vi "poc.ip.kria.vi"(0 "ip.reset":bool, 1 "TDATA":u64, 2 "TKEEP":u8, 3 "TUSER":bool, 4 "TVALID":bool, 5 "TLAST":bool, 6 "DEBUG.TREADY":bool, 7 "CMD.TREADY":bool, 9 "MDEBUG.TREADY":bool) -> ()   [LabVIEW 2020]
uses:
  <vilib>/Platform/TimedLoop/XDataNode/timing_clust.ctl
  <vilib>/Platform/TimedLoop/XDataNode/nitl_modes.ctl
  <vilib>/Platform/TimedLoop/XDataNode/wakeup.ctl
  submodules/Market.Data.Common/fpga/my.network.data.stream.ctl
  submodules/Market.Data.Bats.Parser/fpga/poc.ip.debug.states.ctl
  submodules/Market.Data.Common/fpga/orderbook.command.ctl
  submodules/Market.Data.Common/fpga/orderbook.command.type.ctl
  submodules/Market.Data.Bats.Parser/fpga/poc.ip.axi.write.states.ctl
  <instrlib>/_niInstr/Network/Types/v1/IPv4 Address.ctl
  <instrlib>/_niInstr/Network/Types/v1/MAC Address.ctl
  Ethernet MAC - Custom/Ethernet MAC - Custom.lvclass
  axi_2_eth_raw.ctl
  <vilib>/rvi/DataTransferAndStorage/Container/Common/niFpgaContainerGetUniqueNameForEmu.vi
  <vilib>/rvi/DataTransferAndStorage/Container/Common/niFpgaContainerSetEmuInfo.vi
  <vilib>/rvi/eio/common/nirviEmuReportErrorAndStop.vi
  <vilib>/rvi/Emulation/niFpgaSctlEmulationGetInTimedLoop.vi
  <vilib>/rvi/Emulation/niFpgaEmulationReportErrorSimple.vi
  <vilib>/rvi/Emulation/niFpgaGetClockAttributes.vi
  <vilib>/rvi/Emulation/niFpgaCriticalErrorInLSC.vi
  <vilib>/rvi/Emulation/niFpgaEmulationIsFPGAContextNoSignature.vi
  <vilib>/rvi/errors/niFpgaSetErrorForExecOnDevCompSimple.vi
  <vilib>/rvi/FIFO/Fifo_Resource/nirvififoEmulationSetSize.vi
  <vilib>/rvi/FIFO/Fifo_Resource/nirviFifoEmulationQueueMgr.vi
  <instcachedir>/0/nirviFifoEmulationQueueMgr_E5CAEC123FF24DC58D834DCA3CDAA9B5.lvgen/nirviFifoEmulationQueueMgr_E5CAEC123FF24DC58D834DCA3CDAA9B5_017.vi
  <vilib>/Utility/error.llb/Clear Errors.vi
  <vilib>/rvi/FIFO/Fifo_Resource/nirvififoEmulationCreateLock.vi
  <vilib>/rvi/Emulation/niFpgaProcessEmulError.vi
  <vilib>/rvi/FIFO/Fifo_Resource/nirvififoEmulationObtainLock.vi
  <vilib>/rvi/FIFO/Fifo_Resource/nirvififoEmulationReleaseLock.vi
  <vilib>/rvi/occurrence/nirviWaitOnOccurrenceBase.vi
  <vilib>/rvi/errors/nirviReportUnexpectedCaseInternalError.vi
  <vilib>/rvi/errors/nirviReportUnexpectedCaseInternalError (U32).vi
  <vilib>/rvi/interface/RandomDataEmulation/nirviRandomDataMultiElementFPGAFIFO.vi
  <instcachedir>/0/nirviRandomDataMultiElementFPGAFIFO_3E9965BA1FAD4E7B8DABA31768A09B1F.lvgen/nirviRandomDataMultiElementFPGAFIFO_3E9965BA1FAD4E7B8DABA31768A09B1F_001.vi
  <vilib>/rvi/interface/RandomDataEmulation/niFpgaRandomDataHandleErrors.vi
  <instcachedir>/0/nirviFifoEmulationQueueMgr_E5CAEC123FF24DC58D834DCA3CDAA9B5.lvgen/nirviFifoEmulationQueueMgr_E5CAEC123FF24DC58D834DCA3CDAA9B5_020.vi
  <vilib>/rvi/DataTransferAndStorage/Container/Common/niFpgaContainerExecOnDevCompGetState.vi
  <vilib>/rvi/Memory/Memory_Emulation/niFpgaMemoryEmulationCacheClearOnFirstRun.vi
  <vilib>/rvi/Memory/Memory_Emulation/nirvimemoryEmulationManagerCache_MakeExclusive.vi
  <vilib>/rvi/Memory/Memory_Emulation/niFpgaMemoryEmulationValidateCache.vi
  <vilib>/rvi/Memory/Memory_Emulation/nirvimemoryEmulationManagerCache_InsertValue.vi
  <vilib>/rvi/Memory/Memory_Emulation/nirvimemoryEmulationManagerCache_ReleaseExclusive.vi
  <vilib>/rvi/Memory/Memory_Emulation/nirvimemoryEmulationManagerCache_GetValue.vi
  <vilib>/rvi/Memory/Memory_Emulation/nirvimemoryEmulationManagerCache_SetValue.vi
  <instcachedir>/0/nirviFifoEmulationQueueMgr_E5CAEC123FF24DC58D834DCA3CDAA9B5.lvgen/nirviFifoEmulationQueueMgr_E5CAEC123FF24DC58D834DCA3CDAA9B5_021.vi
  <vilib>/rvi/FIFO/Fifo_Resource/nirvififoEmulationDetermineInputValidOut.vi
  <instcachedir>/0/nirviFifoEmulationQueueMgr_E5CAEC123FF24DC58D834DCA3CDAA9B5.lvgen/nirviFifoEmulationQueueMgr_E5CAEC123FF24DC58D834DCA3CDAA9B5_018.vi
  <vilib>/rvi/Emulation/niFpgaSctlEmulationResourceMgr.vi
  <instrlib>/_niInstr/Network/IPv4/Data Stream/v1/Read IPv4 Header.vi
  <instrlib>/_niInstr/Network/IPv4/UDP/Data Stream/v1/Read End of Bad Frame.vi
  <instrlib>/_niInstr/Network/IPv4/UDP/Data Stream/v1/Read End of Good Frame.vi
  <instrlib>/_niInstr/Network/IPv4/UDP/Data Stream/v1/Read Data Stream.vi
  <vilib>/Platform/TimedLoop/XDataNode/XDataNode.xnode
  <vilib>/rvi/LocalResourceManager/LocalResourceManager.xnode
  <vilib>/rvi/DataTransferAndStorage/Container/XNode/niFpgaContainer.xnode
  <vilib>/rvi/FIFO/Fifo_Resource/nirvififoEmulationRead.vi
  <vilib>/rvi/interface/RandomDataEmulation/nirviRandomDataFpgaMultiElementTemplate.vi
  <vilib>/rvi/DataTransferAndStorage/Register/Emulation/niFpgaRegisterEmulationRefIn.vi
  <vilib>/rvi/FIFO/Fifo_Resource/niFpgaFifoEmulationRefIn.vi
  <vilib>/rvi/Memory/Memory_Emulation/niFpgaMemoryEmulationRefIn.vi
  <vilib>/rvi/FIFO/Fifo_Resource/nirvififoEmulationWrite.vi
  <vilib>/Platform/TimedLoop/XDataNode/XDNodeRunTimeDep.lvlib
  submodules/Market.Data.Common/fpga/fpganow.common.fpga.lvlib
  <instrlib>/_niInstr/Network/IPv4/UDP/Data Stream/v1/niInstr IPv4 UDP Data Stream v1.lvclass
  <instrlib>/_niInstr/Network/Ethernet/Utility/v1/FPGA/niInstr Ethernet Utilities FPGA v1.lvlib
  <instrlib>/_niInstr/Network/IPv4/FPGA/v1/niInstr IPv4 FPGA v1.lvlib
  <instrlib>/_niInstr/Network/IPv4/UDP/FPGA/v1/niInstr IPv4 UDP FPGA v1.lvlib
  <instrlib>/_niInstr/Network/Types/v1/niInstr Network Types v1.lvlib
  <instrlib>/_niInstr/Network/IPv4/Data Stream/v1/niInstr IPv4 Data Stream v1.lvclass
panel:
  out "MDEBUG.TLAST":bool
  out "MDEBUG.TVALID":bool
  out "MDEBUG.TKEEP":u8
  out "MDEBUG.TDATA":u64
  out "CMD.TKEEP":u8
  out "CMD.TDATA":u64
  out "CMD.TLAST":bool
  out "CMD.TVALID":bool
  out "DEBUG.TLAST":bool
  out "DEBUG.TVALID":bool
  out "DEBUG.TKEEP":u8
  out "DEBUG.TDATA":u64
  # "This VI will be IP Exported"
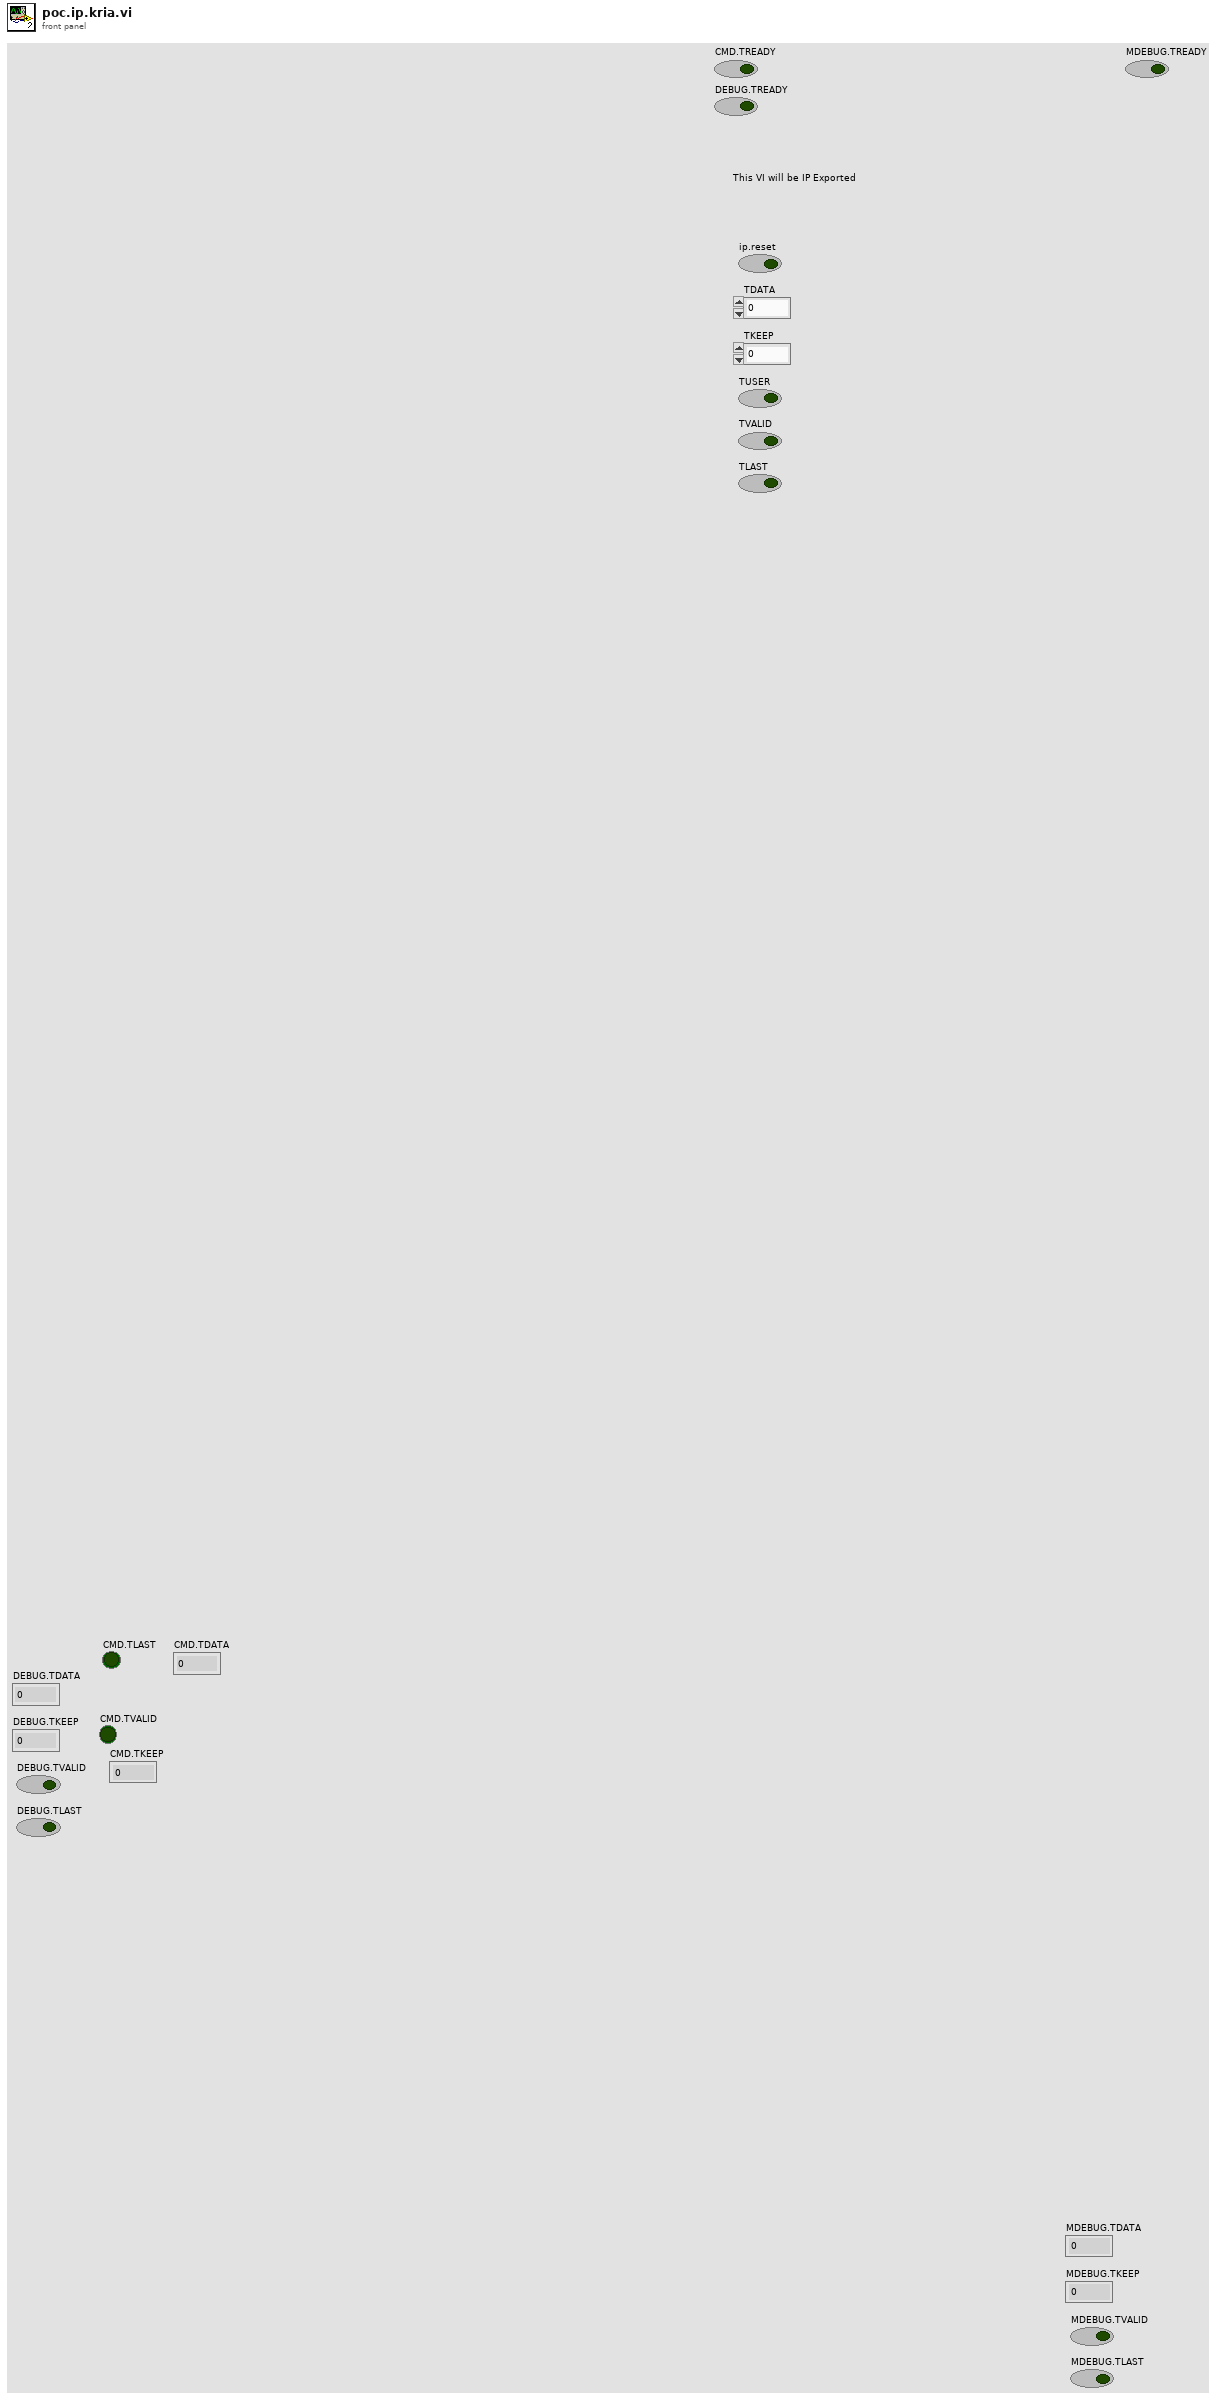
[diagram p1: front panel]
types:
  T1 = typedef "XDNodeRunTimeDep.lvlib/timing_clust.ctl" = cluster{"Expected End [f-1]":u64, "Actual End [f-1]":u64, "Finished Late? [f-1]":bool, "Expected End [i-1]":u64, "Actual End [i-1]":u64, "Finished Late? [i-1]":bool, "Expected Start [i]":u64, "Actual Start [i]":u64, "Expected Start [f]":u64, "Actual Start [f]":u64, "Source Name":string, "Structure Name":string, "Period":i64, "Deadline":i64, "Offset":i64, "Start":i64, "Priority":i32, "Timeout":i32, "Mode":T2, "Wakeup Reason":T3, "Error":errorcluster, "Source Type":string, "Secondary Source Type":string, "Global End Time":u64, "Global Start Time":u64, "Frame Duration":u64, "Iteration Duration":u64, "Assigned CPU":i32, "I/O Scan Engine Mode":u32}
  T2 = typedef "XDNodeRunTimeDep.lvlib/nitl_modes.ctl" = enum32{"No Change", "Process missed periods, maintain original phase", "Discard missed periods, maintain original phase", "Process missed periods, ignore original phase", "Discard missed periods, ignore original phase"}
  T3 = typedef "XDNodeRunTimeDep.lvlib/wakeup.ctl" = enum32{"Normal", "Aborted", "Asynchronous wakeup", "Timing source error", "Timed loop error", "Timeout"}
  T4 = typedef "niInstr Network Types v1.lvlib/MAC Address.ctl" = u8[]
  T5 = typedef "niInstr Network Types v1.lvlib/IPv4 Address.ctl" = u8[]
  T6 = typedef "my.network.data.stream.ctl" = cluster{"data":u8[], "data valid":bool, "byte enables":bool[], "eof.good":bool, "eof.bad":bool, "frame.start":u64}
  T7 = cluster{"TDATA":u64, "TKEEP":u8, "TVALID":bool, "TLAST":bool, "TUSER":bool}
  T8 = cluster{"data valid":bool, "end.of.frame":bool, "start.of.frame":bool, "data":u64, "byte enables":u8}
  T9 = typedef "axi_2_eth_raw.ctl" = cluster{"data valid":bool, "end.of.frame":bool, "start.of.frame":bool, "data":u64, "byte enables":u8}
  T10 = typedef "niInstr IPv4 FPGA v1.lvlib/IPv4 Header.ctl" = cluster{"Version":fxp<+,4,4>, "IHL":fxp<+,4,4>, "DSCP":fxp<+,6,6>, "ECN":fxp<+,2,2>, "Total Length":u16, "Identification":u16, "Flags":fxp<+,3,3>, "Fragment Offset":fxp<+,13,13>, "Time To Live":u8, "Protocol":T11, "Header Checksum":u16, "Source IP":u8[], "Dest IP":u8[]}
  T11 = typedef "niInstr IPv4 FPGA v1.lvlib/IPv4 Protocols.ctl" = u8
  T12 = typedef "niInstr Ethernet Utilities FPGA v1.lvlib/Network Data Stream.ctl" = cluster{"data":u8[], "data valid":bool, "byte enables":bool[]}
  T13 = typedef "poc.ip.debug.states.ctl" = enum16{"Wait", "Write.Data"}
  T14 = typedef "poc.ip.axi.write.states.ctl" = enum16{"Wait", "Collect"}
  T15 = typedef "fpganow.common.fpga.lvlib/orderbook.command.ctl" = cluster{"type":T16, "side":u8, "orderId ":u64, "quantity":u32, "symbol":u64, "price":u64, "executed.qty":u32, "canceled.qty":u32, "remaining.qty":u32, "seconds":u64, "nanoseconds":u64, "Add":bool, "Edit":bool, "Remove":bool, "seq no":u32, "recv.time":u64, "parse.time":u64}
  T16 = typedef "fpganow.common.fpga.lvlib/orderbook.command.type.ctl" = enum8{"Time", "AddOrder", "OrderExecuted", "OrderExecutedAtPrice", "ReduceSize", "ModifyOrder", "DeleteOrder", "Get.Everything", "Get.All.Orders", "Get.Top"}
  T17 = cluster{"state":T13, "ob.cmd":T15, "index":i16, "TLAST":bool, "TDATA":u64}
  T18 = cluster{"state":T13, "arr":u64[], "index":u8, "TLAST":bool, "TDATA":u64}
  T19 = cluster{"type":enum8{"Time", "AddOrder", "OrderExecuted", "OrderExecutedAtPrice", "ReduceSize", "ModifyOrder", "DeleteOrder", "Get.Everything", "Get.All.Orders", "Get.Top"}, "side":u8, "orderId ":u64, "quantity":u32, "symbol":u64, "price":u64, "executed.qty":u32, "canceled.qty":u32, "remaining.qty":u32, "seconds":u64, "nanoseconds":u64, "Add":bool, "Edit":bool, "Remove":bool, "seq no":u32, "recv.time":u64, "parse.time":u64}
  T20 = enum8{"Time", "AddOrder", "OrderExecuted", "OrderExecutedAtPrice", "ReduceSize", "ModifyOrder", "DeleteOrder", "Get.Everything", "Get.All.Orders", "Get.Top"}
  T21 = cluster{"data":u8[], "data valid":bool, "byte enables":bool[], "eof.good":bool, "eof.bad":bool, "Timestamp":u64}
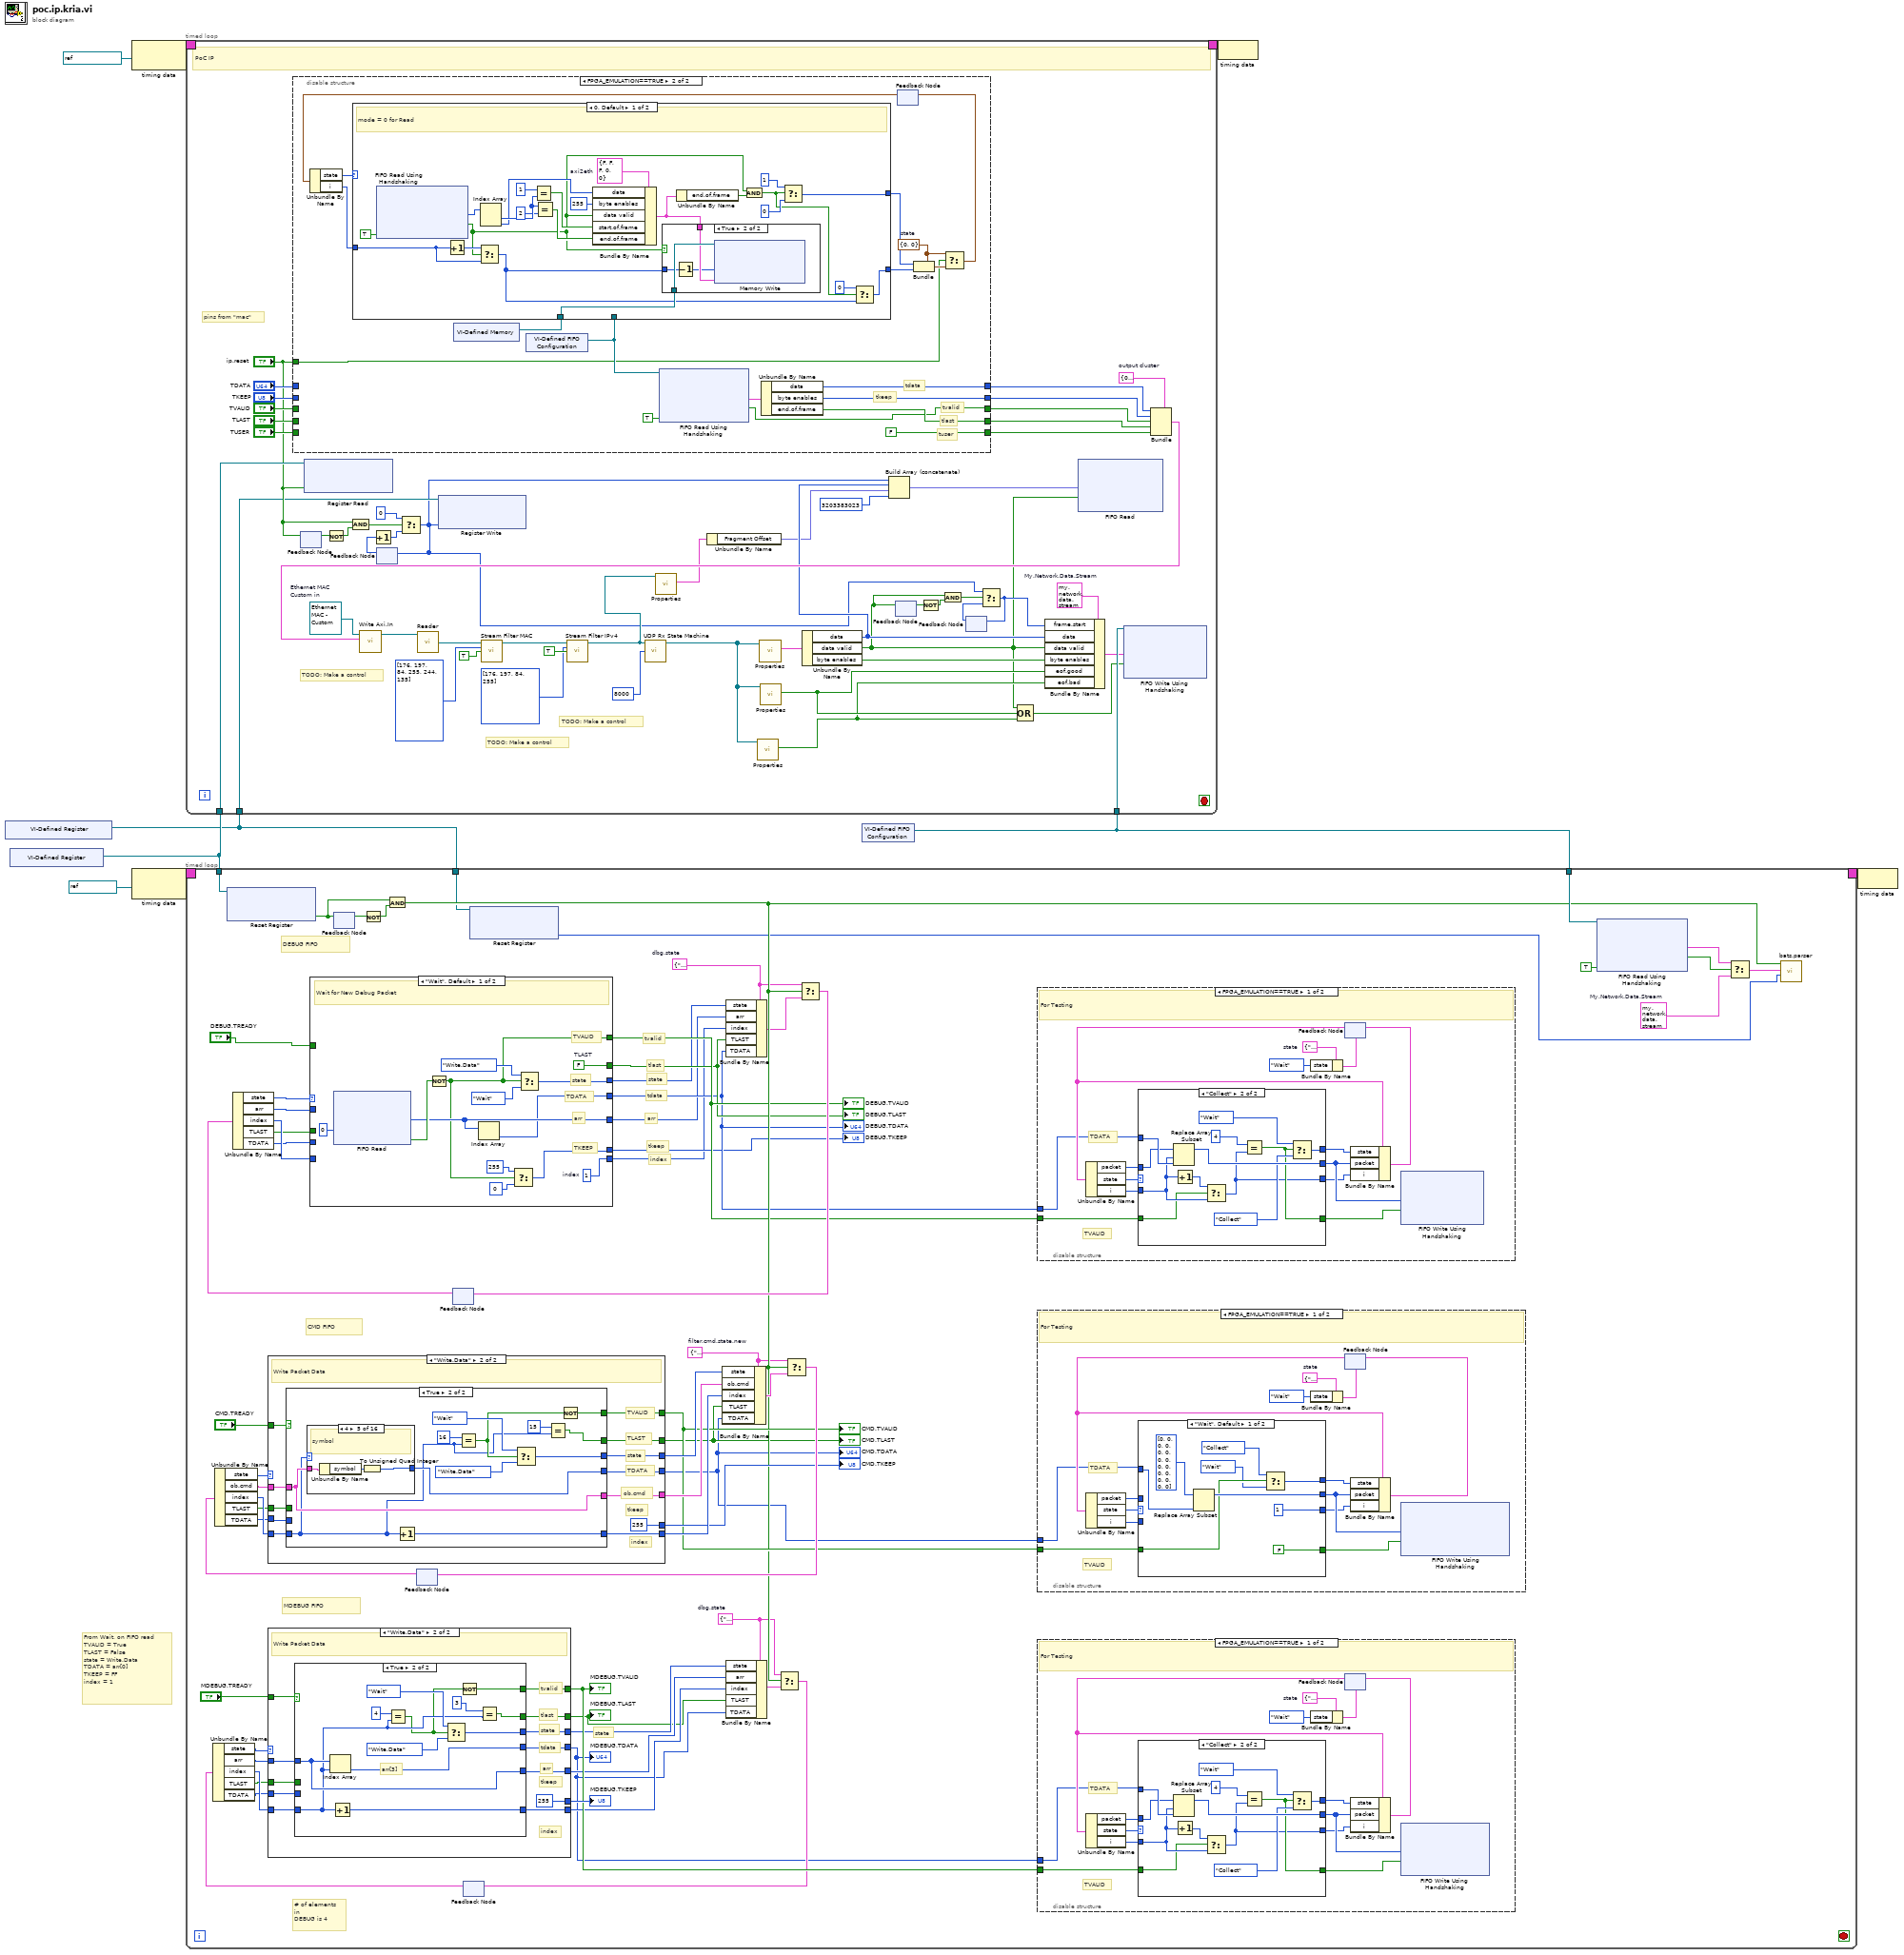
[diagram p0: block diagram]
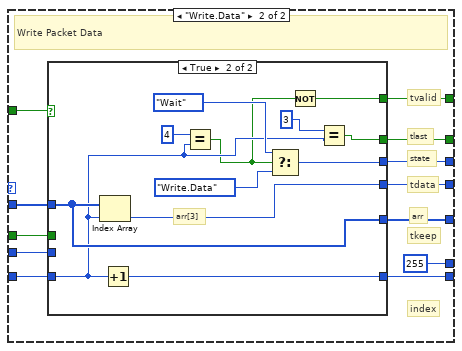
[diagram p2: hidden frame]
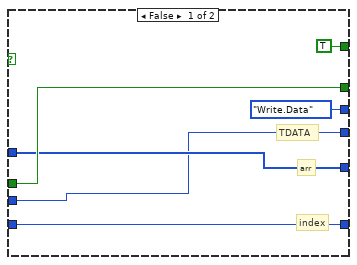
[diagram p3: hidden frame]
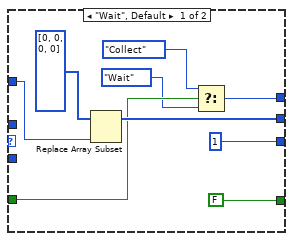
[diagram p4: hidden frame]
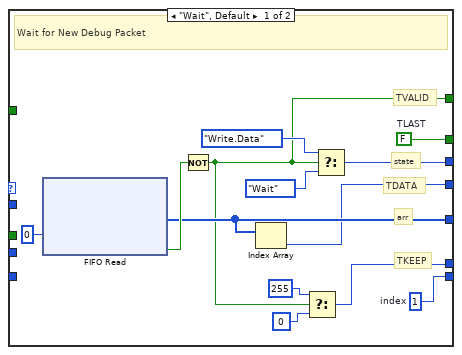
[diagram p6: hidden frame]
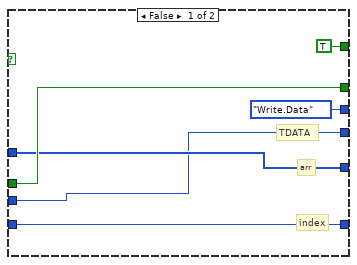
[diagram p7: hidden frame]
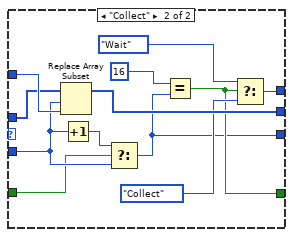
[diagram p8: hidden frame]
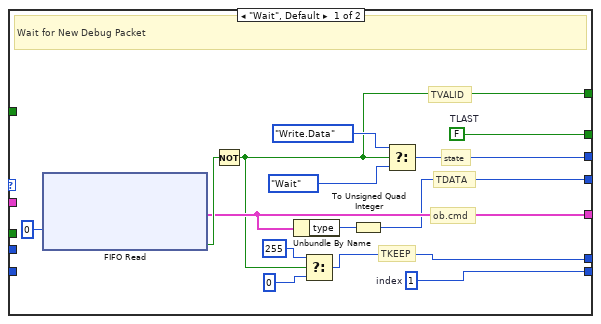
[diagram p10: hidden frame]
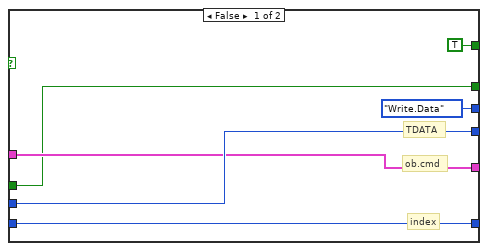
[diagram p11: hidden frame]
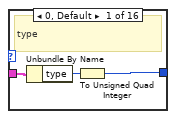
[diagram p12: hidden frame]
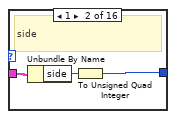
[diagram p13: hidden frame]
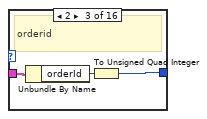
[diagram p14: hidden frame]
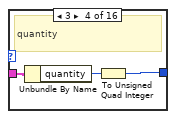
[diagram p15: hidden frame]
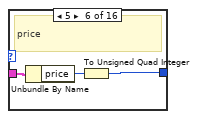
[diagram p16: hidden frame]
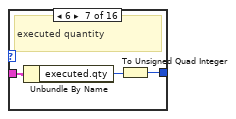
[diagram p17: hidden frame]
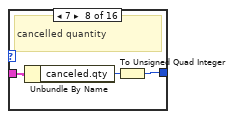
[diagram p18: hidden frame]
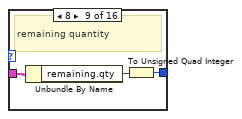
[diagram p19: hidden frame]
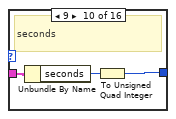
[diagram p20: hidden frame]
diagram:
  # "From Wait, on FIFO read\nTVALID = True\nTLAST = False\nstate = Write.Data\nTDATA = arr[0]\nTKEEP = FF\nindex = 1"
  n1 = xnode "VI-Defined Register"() -> ("Register Out"=w1:refnum<k21>)
  n2 = xnode "VI-Defined Register"() -> ("Register Out"=w2:refnum<k21>)
  n3 = node-c288(refnum<k21> "156.28MHz" ("Source Name")) -> (w9:T1)
  n4 = node-c288(refnum<k21> "100MHz" ("Source Name")) -> (w6:T1)
  n5 = xnode "VI-Defined FIFO Configuration"() -> ("FIFO Out"=w3:refnum<k21>)
  n6 = timed-loop {
    timing: w9 -> [_]
    timing-out: [_] -> w8
    tunnel: w3 -> [w39]
    tunnel: w2 -> [w36]
    tunnel: w1 -> [w27]
    stop <- _ stop-if-true
    w40 = T6 {"data"=[0, 0, 0, 0, 0, 0, 0, 0], "data valid"=FALSE, "byte enables"=[FALSE, FALSE, FALSE, FALSE, FALSE, FALSE, FALSE, FALSE], "eof.good"=FALSE, "eof.bad"=FALSE, "frame.start"=0}  # My.Network.Data.Stream
    w47 = refnum<class "Ethernet MAC - Custom.lvclass"> refnum  # Ethernet MAC Custom in
    w56 = T7 {"TDATA"=0, "TKEEP"=0, "TVALID"=FALSE, "TLAST"=FALSE, "TUSER"=FALSE}  # output cluster
    # "pins from \"mac\""
    # "TODO: Make a control"
    # "TODO: Make a control"
    # "TODO: Make a control"
    # "PoC IP"
    n7 = disable-structure shown="FPGA_EMULATION==TRUE" {
      disable-tunnel: [w66 w70] -> w46
      disable-tunnel: "TDATA" -> [w66 _]
      disable-tunnel: [w65 w69] -> w45
      disable-tunnel: "TKEEP" -> [w65 _]
      disable-tunnel: [w64 w67] -> w44
      disable-tunnel: "TVALID" -> [w64 _]
      disable-tunnel: [w63 w71] -> w43
      disable-tunnel: "TLAST" -> [w63 _]
      disable-tunnel: [w62 FALSE ("TUSER")] -> w32
      disable-tunnel: "TUSER" -> [w62 _]
      disable-tunnel: "ip.reset" -> [_ w68]
      frame condition #0 {
      }
      frame condition #1 (active) {
        w80 = cluster{"state":u8, "i":u16} {"state"=0, "i"=0}  # state
        # "tkeep"
        # "tdata"
        # "tuser"
        # "tlast"
        # "tvalid"
        n8 = xnode "VI-Defined Memory"() -> ("Memory Out"=w76:refnum<k21>)
        n9 = xnode "VI-Defined FIFO Configuration"() -> ("FIFO Out"=w73:refnum<k21>)
        n10 = xnode "FIFO Read Using Handshaking"("Ready for Output"=TRUE, "FIFO In"=w73) -> ("Element"=w74:T8, "Output Valid"=w67:bool)  [unwired: 1 out]
        n11 = Unbundle By Name(w74) -> ("data"=w70:u64, "byte enables"=w69:u8, "end.of.frame"=w71:bool)
        n12 = feedback #1() -> (w82:cluster{"state":u8, "i":u16})  [unwired: 1 in]
        n13 = Unbundle By Name(w82) -> ("state"=w83:u8, "i"=w84:u16)
        n14 = case shown="0, Default" w83 {
          tunnel: w84 -> [w96 w113]
          tunnel: w76 -> [w95 w125]
          tunnel: [w89 w119] -> w78
          tunnel: [w90 w122] -> w77
          tunnel: w73 -> [_ w112]
          frame 0, Default {
            w107 = T9 {"data valid"=FALSE, "end.of.frame"=FALSE, "start.of.frame"=FALSE, "data"=0, "byte enables"=0}  # axi2eth
            # "mode = 0 for Read"
            n15 = xnode "FIFO Read Using Handshaking"("Ready for Output"=TRUE) -> ("Element"=w106:u64[], "Output Valid"=w85:bool)  [unwired: 1 in, 1 out]
            n16 = Increment(x=w96) -> (x+1=w97:u16)
            n17 = Select(t=w97, s=w85, f=w96) -> (s? t:f=w88:u16)
            n18 = Index Array(array=w106) -> (element #1=w105:u64, element #2=w99:u64)  [unwired: 2 in]
            n19 = Equal?(x=u64 1, y=w105) -> (x = y?=w101:bool)
            n20 = Equal?(x=w105, y=u64 2) -> (x = y?=w102:bool)
            n21 = Bundle By Name(cluster=w107, "data"=w99, "byte enables"=u8 255 ("number"), "data valid"=w85, "start.of.frame"=w101, "end.of.frame"=w102) -> (w94:T9)
            n22 = case shown="True" w85 {
              tunnel: w95 -> [_ w111]
              tunnel: w94 -> [_ w110]
              tunnel: w88 -> [_ w109]
              frame False {
              }
              frame True {
                n23 = Decrement(x=w109) -> (x-1=w108:u16)
                n24 = xnode "Memory Write"("Address"=w108, "Data"=w110, "Memory In"=w111) -> ()  [unwired: 1 out]
              }
            }
            n25 = Unbundle By Name(w94) -> ("end.of.frame"=w93:bool)
            n26 = And(x=w85, y=w93) -> (x .and. y?=w87:bool)
            n27 = Select(t=u8 1, s=w87, f=u8 0 ("t")) -> (s? t:f=w90:u8)
            n28 = Select(t=u16 0, s=w87, f=w88) -> (s? t:f=w89:u16)
          }
          frame 1 {
            # "mode = 1 for Write"
            n29 = xnode "Memory Read"("Address"=w113, "Memory In"=w125) -> ("Data"=w124:T8)  [unwired: 1 out]
            n30 = feedback-in #2(w124) -> ()
            n31 = feedback #2() -> (w114:T8)  [unwired: 1 in]
            n32 = feedback-in #3(TRUE ("Input Valid")) -> ()
            n33 = feedback #3(FALSE ("Input Valid")) -> (w115:bool)
            n34 = Increment(x=w113) -> (x+1=w119:u16)
            n35 = Unbundle By Name(w114) -> ("end.of.frame"=w123:bool)
            n36 = xnode "FIFO Write Using Handshaking"("Element"=w114, "Input Valid"=w115, "FIFO In"=w112) -> ()  [unwired: 2 out]
            n37 = And(x=w123, y=w115) -> (x .and. y?=w116:bool)
            n38 = Select(t=u8 0 ("f"), s=w116, f=u8 1) -> (s? t:f=w122:u8)
          }
        }
        n39 = Bundle(cluster=w80, "state"=w77, "i"=w78) -> (w79:cluster{"state":u8, "i":u16})
        n40 = Select(t=w80, s=w68, f=w79) -> (s? t:f=w81:cluster{"state":u8, "i":u16})
        n41 = feedback-in #1(w81) -> ()
      }
    }
    n42 = feedback #4() -> (w31:bool)  [unwired: 1 in]
    n43 = feedback-in #4("ip.reset") -> ()
    n44 = xnode "Register Read"("Data"="ip.reset", "Register In"=w36) -> ()  [unwired: 1 out]
    n45 = Not(x=w31) -> (.not. x?=w30:bool)
    n46 = And(x="ip.reset", y=w30) -> (x .and. y?=w28:bool)
    n47 = feedback #5() -> (w25:u64)  [unwired: 1 in]
    n48 = Increment(x=w25) -> (x+1=w24:u64)
    n49 = Select(t=u64 0, s=w28, f=w24) -> (s? t:f=w10:u64)
    n50 = feedback-in #5(w10) -> ()
    n51 = xnode "Register Write"("Data"=w10, "Register In"=w27) -> ()  [unwired: 1 out]
    n52 = feedback #6() -> (w14:bool)  [unwired: 1 in]
    n53 = Not(x=w14) -> (.not. x?=w13:bool)
    n54 = feedback #7() -> (w16:u64)  [unwired: 1 in]
    n55 = Bundle(cluster=w56, "TDATA"=w46, "TKEEP"=w45, "TVALID"=w44, "TLAST"=w43, "TUSER"=w32) -> (w42:T7)
    n56 = call-dynamic "Write Axi.In.vi"("Axi.In"=w42, "Ethernet MAC - Custom in"=w47) -> ("Ethernet MAC - Custom out"=w54:refnum<class "Ethernet MAC - Custom.lvclass">)  [unwired: 8 in, 1 out]
    n57 = call-dynamic "Reader.vi"("Ethernet MAC - Custom.lvclass"=w54) -> ("niInstr Ethernet MAC Raw Stream v1.lvclass"=w55:refnum<class "niInstr Ethernet MAC Raw Stream v1.lvclass">)  [unwired: 13 in, 1 out]
    n58 = call <instrlib>:"Stream Filter MAC.vi"("niInstr Ethernet MAC Raw Stream v1 in"=w55, "MAC Address"=T4 [176, 197, 84, 255, 244, 135], "Promiscuous?"=TRUE) -> ("niInstr Ethernet MAC Data Stream v1 out"=w48:refnum<class "niInstr Ethernet MAC Data Stream v1.lvclass">)  [unwired: 12 in]
    n59 = call <instrlib>:"Stream Filter IPv4.vi"("niInstr Ethernet MAC Data Stream v1 in"=w48, "IP Address"=T5 [176, 197, 84, 255], "disable IP filtering"=TRUE) -> ("niInstr IPv4 Data Stream out"=w20:refnum<class "niInstr IPv4 Data Stream v1.lvclass">)  [unwired: 12 in]
    n60 = call <instrlib>:"UDP Rx State Machine.vi"("niInstr IPv4 Data Stream in"=w20, "Dest Port"=u16 8000) -> ("niInstr IPv4 UDP Data Stream out"=w21:refnum<class "niInstr IPv4 UDP Data Stream v1.lvclass">)  [unwired: 13 in]
    n61 = call-poly <instrlib>:"Properties.vi"("niInstr IPv4 Data Stream in"=w20) -> ("IPv4 Header"=w19:T10)  [unwired: 9 in, 1 out]
    n62 = Unbundle By Name(w19) -> ("Fragment Offset"=w18:fxp<+,13,13>)
    n63 = call-poly <instrlib>:"Properties.vi"("niInstr IPv4 UDP Data Stream in"=w21) -> ("End of Bad Frame"=w33:bool)  [unwired: 9 in, 1 out]
    n64 = call-poly <instrlib>:"Properties.vi"("niInstr IPv4 UDP Data Stream v1.lvclass"=w21) -> ("Data Stream"=w41:T12)  [unwired: 9 in, 1 out]
    n65 = call-poly <instrlib>:"Properties.vi"("niInstr IPv4 UDP Data Stream in"=w21) -> ("End of Good Frame"=w34:bool)  [unwired: 9 in, 1 out]
    n66 = Unbundle By Name(w41) -> ("data"=w22:u8[], "data valid"=w11:bool, "byte enables"=w35:bool[])
    n67 = Build Array (concatenate)(w10, w22, w18, u64 3203383023 ("element")) -> (w23:fxp<+,64,64>[])
    n68 = feedback-in #6(w11) -> ()
    n69 = And(x=w11, y=w13) -> (x .and. y?=w12:bool)
    n70 = Select(t=w10, s=w12, f=w16) -> (s? t:f=w15:u64)
    n71 = feedback-in #7(w15) -> ()
    n72 = Compound Arithmetic op=OR(w11, w34, w33) -> (w37:bool)
    n73 = Bundle By Name(cluster=w40, "frame.start"=w15, "data"=w22, "data valid"=w11, "byte enables"=w35, "eof.good"=w34, "eof.bad"=w33) -> (w38:T6)
    n74 = xnode ("FIFO Read")("Element"=w23, "Input Valid"=w11) -> ()  [unwired: 1 in, 2 out]
    n75 = xnode "FIFO Write Using Handshaking"("Element"=w38, "Input Valid"=w37, "FIFO In"=w39) -> ()  [unwired: 2 out]
  }
  n76 = timed-loop {
    timing: w6 -> [_]
    timing-out: [_] -> w5
    tunnel: w2 -> [w191]
    tunnel: w3 -> [w174]
    tunnel: w1 -> [w159]
    stop <- _ stop-if-true
    w160 = T17 {"state"=enum."Wait", "ob.cmd"={"type"=enum."AddOrder", "side"=0, "orderId "=0, "quantity"=0, "symbol"=0, "price"=0, "executed.qty"=0, "canceled.qty"=0, "remaining.qty"=0, "seconds"=0, "nanoseconds"=0, "Add"=FALSE, "Edit"=FALSE, "Remove"=FALSE, "seq no"=0, "recv.time"=0, "parse.time"=0}, "index"=0, "TLAST"=FALSE, "TDATA"=0}  # filter.cmd.state.new
    w154 = T18 {"state"=enum."Wait", "arr"=[0, 0, 0, 0], "index"=0, "TLAST"=FALSE, "TDATA"=0}  # dbg.state
    w169 = T6 {"data"=[0, 0, 0, 0, 0, 0, 0, 0], "data valid"=FALSE, "byte enables"=[FALSE, FALSE, FALSE, FALSE, FALSE, FALSE, FALSE, FALSE], "eof.good"=FALSE, "eof.bad"=FALSE, "frame.start"=0}  # My.Network.Data.Stream
    w147 = T18 {"state"=enum."Wait", "arr"=[0, 0, 0, 0], "index"=0, "TLAST"=FALSE, "TDATA"=0}  # dbg.state
    # "index"
    # "tkeep"
    # "arr"
    # "tdata"
    # "state"
    # "tlast"
    # "tvalid"
    # "state"
    # "# of elements \nin \nDEBUG is 4"
    # "MDEBUG FIFO"
    # "DEBUG FIFO"
    # "CMD FIFO"
    n77 = xnode "Reset Register"("Register In"=w191) -> ("Data"=w175:bool)  [unwired: 1 out]
    n78 = feedback-in #8(w175) -> ()
    n79 = feedback #8() -> (w177:bool)  [unwired: 1 in]
    n80 = Not(x=w177) -> (.not. x?=w176:bool)
    n81 = And(x=w175, y=w176) -> (x .and. y?=w161:bool)
    n82 = feedback #9() -> (w183:T17)  [unwired: 1 in]
    n83 = Unbundle By Name(w183) -> ("state"=w182:T13, "ob.cmd"=w181:T15, "index"=w180:i16, "TLAST"=w143:bool, "TDATA"=w142:u64)
    n84 = case shown="\"Write.Data\"" w182 {
      tunnel: [w360 w371] -> w186
      tunnel: w180 -> [_ w366]
      tunnel: [w361 w369] -> w188
      tunnel: [w354 w365] -> w185
      tunnel: w181 -> [_ w368]
      tunnel: [w352 w367] -> w144
      tunnel: [w351 u8 255 ("DEBUG.TKEEP")] -> w179
      tunnel: [w359 w370] -> w145
      tunnel: [w349 w372] -> w178
      tunnel: w143 -> [_ w362]
      tunnel: w142 -> [_ w363]
      tunnel: "CMD.TREADY" -> [_ w364]
      frame "Wait", Default {
        w359 = FALSE  # TLAST
        w360 = i16 1  # index
        # "ob.cmd"
        # "TKEEP"
        # "TDATA"
        # "state"
        # "TVALID"
        # "Wait for New Debug Packet"
        n85 = xnode ("FIFO Read")("Timeout"=0) -> ("Element"=w354:T19, "Timed Out?"=w355:bool)  [unwired: 1 in, 1 out]
        n86 = Not(x=w355) -> (.not. x?=w349:bool)
        n87 = Unbundle By Name(w354) -> ("type"=w353:T20)
        n88 = Select(t=u8 255 ("DEBUG.TKEEP"), s=w349, f=u8 0 ("DEBUG.TKEEP")) -> (s? t:f=w351:u8)
        n89 = To Unsigned Quad Integer(1:w353) -> (0:w352:u64)
        n90 = Select(t=poc.ip.debug.states."Write.Data", s=w349, f=poc.ip.debug.states."Wait") -> (s? t:f=w361:T13)
      }
      frame "Write.Data" {
        # "index"
        # "tkeep"
        # "ob.cmd"
        # "TDATA"
        # "state"
        # "TLAST"
        # "TVALID"
        # "Write Packet Data"
        n91 = case shown="True" w364 {
          tunnel: [TRUE w383] -> w372
          tunnel: [w375 w391] -> w371
          tunnel: [w374 w380] -> w370
          tunnel: [poc.ip.debug.states."Write.Data" w389] -> w369
          tunnel: w366 -> [w375 w382]
          tunnel: w368 -> [w376 w385]
          tunnel: [w377 w386] -> w367
          tunnel: [w376 w385] -> w365
          tunnel: w363 -> [w377 _]
          tunnel: w362 -> [w374 _]
          frame False {
            # "TDATA"
            # "ob.cmd"
            # "index"
          }
          frame True {
            n92 = case shown="4" w382 {
              tunnel: w385 -> [w394 w397 w400 w403 w406 w409 w412 w415 w418 w421 w424 w427 w430 w432 w435 _]
              tunnel: [w392 w395 w398 w401 w404 w407 w410 w413 w416 w419 w422 w425 w428 w433 w436 w438] -> w386
              frame 0, Default {
                # "type"
                n93 = Unbundle By Name(w394) -> ("type"=w393:T16)
                n94 = To Unsigned Quad Integer(1:w393) -> (0:w392:u64)
              }
              frame 1 {
                # "side"
                n95 = Unbundle By Name(w397) -> ("side"=w396:u8)
                n96 = To Unsigned Quad Integer(1:w396) -> (0:w395:u64)
              }
              frame 2 {
                # "orderid"
                n97 = Unbundle By Name(w400) -> ("orderId"=w399:u64)
                n98 = To Unsigned Quad Integer(1:w399) -> (0:w398:u64)
              }
              frame 3 {
                # "quantity"
                n99 = Unbundle By Name(w403) -> ("quantity"=w402:u32)
                n100 = To Unsigned Quad Integer(1:w402) -> (0:w401:u64)
              }
              frame 4 {
                # "symbol"
                n101 = Unbundle By Name(w406) -> ("symbol"=w405:u64)
                n102 = To Unsigned Quad Integer(1:w405) -> (0:w404:u64)
              }
              frame 5 {
                # "price"
                n103 = Unbundle By Name(w409) -> ("price"=w408:u64)
                n104 = To Unsigned Quad Integer(1:w408) -> (0:w407:u64)
              }
              frame 6 {
                # "executed quantity"
                n105 = Unbundle By Name(w412) -> ("executed.qty"=w411:u32)
                n106 = To Unsigned Quad Integer(1:w411) -> (0:w410:u64)
              }
              frame 7 {
                # "cancelled quantity"
                n107 = Unbundle By Name(w415) -> ("canceled.qty"=w414:u32)
                n108 = To Unsigned Quad Integer(1:w414) -> (0:w413:u64)
              }
              frame 8 {
                # "remaining quantity"
                n109 = Unbundle By Name(w418) -> ("remaining.qty"=w417:u32)
                n110 = To Unsigned Quad Integer(1:w417) -> (0:w416:u64)
              }
              frame 9 {
                # "seconds"
                n111 = Unbundle By Name(w421) -> ("seconds"=w420:u64)
                n112 = To Unsigned Quad Integer(1:w420) -> (0:w419:u64)
              }
              frame 10 {
                # "nanoseconds"
                n113 = Unbundle By Name(w424) -> ("nanoseconds"=w423:u64)
                n114 = To Unsigned Quad Integer(1:w423) -> (0:w422:u64)
              }
              frame 11 {
                # "type"
                n115 = call "ser.bools.vi"("orderbook.command"=w427) -> ("Numeric"=w426:u32)  [unwired: 10 in]
                n116 = To Unsigned Quad Integer(1:w426) -> (0:w425:u64)
              }
              frame 12 {
                # "sequence no"
                n117 = Unbundle By Name(w430) -> ("seq no"=w429:u32)
                n118 = To Unsigned Quad Integer(1:w429) -> (0:w428:u64)
              }
              frame 13 {
                # "recv.time"
                n119 = Unbundle By Name(w432) -> ("recv.time"=w431:u64)
                n120 = To Unsigned Quad Integer(1:w431) -> (0:w433:u64)
              }
              frame 14 {
                # "parse.time"
                n121 = Unbundle By Name(w435) -> ("parse.time"=w434:u64)
                n122 = To Unsigned Quad Integer(1:w434) -> (0:w436:u64)
              }
              frame 15 {
                # "Reserved for Filter time"
                n123 = To Unsigned Quad Integer(1:u64 3735928559 ("number")) -> (0:w438:u64)
              }
            }
            n124 = Increment(x=w382) -> (x+1=w391:i16)
            n125 = Equal?(x=i16 16, y=w382) -> (x = y?=w384:bool)
            n126 = Select(t=poc.ip.debug.states."Wait", s=w384, f=poc.ip.debug.states."Write.Data") -> (s? t:f=w389:T13)
            n127 = Equal?(x=i16 15, y=w382) -> (x = y?=w380:bool)
            n128 = Not(x=w384) -> (.not. x?=w383:bool)
          }
        }
      }
    }
    "CMD.TVALID" <- w178
    "CMD.TLAST" <- w145
    "CMD.TDATA" <- w144
    "CMD.TKEEP" <- w179
    n129 = feedback #10() -> (w189:T18)  [unwired: 1 in]
    n130 = Unbundle By Name(w189) -> ("state"=w132:T13, "arr"=w131:u64[], "index"=w130:u8, "TLAST"=w128:bool, "TDATA"=w129:u64)
    n131 = case shown="\"Wait\", Default" w132 {
      tunnel: [w192 w212] -> w134
      tunnel: w130 -> [_ w216]
      tunnel: [w204 w210] -> w138
      tunnel: [w198 w206] -> w136
      tunnel: w131 -> [_ w209]
      tunnel: [w197 w215] -> w137
      tunnel: [w194 u8 255 ("DEBUG.TKEEP")] -> w135
      tunnel: [w203 w211] -> w139
      tunnel: [w193 w213] -> w140
      tunnel: "DEBUG.TREADY" -> [_ w208]
      tunnel: w128 -> [_ w207]
      tunnel: w129 -> [_ w205]
      frame "Wait", Default {
        w203 = FALSE  # TLAST
        w192 = u8 1  # index
        # "TKEEP"
        # "arr"
        # "TDATA"
        # "TVALID"
        # "state"
        # "Wait for New Debug Packet"
        n132 = xnode ("FIFO Read")("Timeout"=0) -> ("Element"=w198:u64[], "Timed Out?"=w199:bool)  [unwired: 1 in, 1 out]
        n133 = Not(x=w199) -> (.not. x?=w193:bool)
        n134 = Index Array(array=w198) -> (element=w197:u64)  [unwired: 1 in]
        n135 = Select(t=u8 255 ("DEBUG.TKEEP"), s=w193, f=u8 0 ("DEBUG.TKEEP")) -> (s? t:f=w194:u8)
        n136 = Select(t=poc.ip.debug.states."Write.Data", s=w193, f=poc.ip.debug.states."Wait") -> (s? t:f=w204:T13)
      }
      frame "Write.Data" {
        # "arr"
        # "tkeep"
        # "tdata"
        # "state"
        # "tlast"
        # "tvalid"
        # "index"
        # "Write Packet Data"
        n137 = case shown="True" w208 {
          tunnel: w216 -> [w219 w225]
          tunnel: [w217 w234] -> w215
          tunnel: [TRUE w223] -> w213
          tunnel: [w219 w226] -> w212
          tunnel: [w221 w228] -> w211
          tunnel: [poc.ip.debug.states."Write.Data" w233] -> w210
          tunnel: w209 -> [w218 w229]
          tunnel: w207 -> [w221 _]
          tunnel: [w218 w229] -> w206
          tunnel: w205 -> [w217 _]
          frame False {
            # "index"
            # "arr"
            # "TDATA"
          }
          frame True {
            # "arr[3]"
            n138 = Index Array(array=w229, index=w225) -> (element=w234:u64)
            n139 = Increment(x=w225) -> (x+1=w226:u8)
            n140 = Equal?(x=u8 4, y=w225) -> (x = y?=w224:bool)
            n141 = Select(t=poc.ip.debug.states."Wait", s=w224, f=poc.ip.debug.states."Write.Data") -> (s? t:f=w233:T13)
            n142 = Not(x=w224) -> (.not. x?=w223:bool)
            n143 = Equal?(x=u8 3, y=w225) -> (x = y?=w228:bool)
          }
        }
      }
    }
    "DEBUG.TDATA" <- w137
    "DEBUG.TKEEP" <- w135
    "DEBUG.TVALID" <- w140
    "DEBUG.TLAST" <- w139
    n144 = feedback #11() -> (w165:T18)  [unwired: 1 in]
    n145 = Unbundle By Name(w165) -> ("state"=w164:T13, "arr"=w163:u64[], "index"=w162:u8, "TLAST"=w156:bool, "TDATA"=w155:u64)
    n146 = case shown="\"Write.Data\"" w164 {
      tunnel: [w270 w290] -> w151
      tunnel: w162 -> [_ w294]
      tunnel: [w282 w288] -> w153
      tunnel: [w276 w284] -> w152
      tunnel: w163 -> [_ w287]
      tunnel: [w275 w293] -> w149
      tunnel: [w272 u8 255 ("DEBUG.TKEEP")] -> w168
      tunnel: [w281 w289] -> w150
      tunnel: [w271 w291] -> w167
      tunnel: "MDEBUG.TREADY" -> [_ w286]
      tunnel: w156 -> [_ w285]
      tunnel: w155 -> [_ w283]
      frame "Wait", Default {
        w281 = FALSE  # TLAST
        w270 = u8 1  # index
        # "TKEEP"
        # "arr"
        # "TDATA"
        # "TVALID"
        # "state"
        # "Wait for New Debug Packet"
        n147 = xnode ("FIFO Read")("Timeout"=0) -> ("Element"=w276:u64[], "Timed Out?"=w277:bool)  [unwired: 1 in, 1 out]
        n148 = Not(x=w277) -> (.not. x?=w271:bool)
        n149 = Index Array(array=w276) -> (element=w275:u64)  [unwired: 1 in]
        n150 = Select(t=u8 255 ("DEBUG.TKEEP"), s=w271, f=u8 0 ("DEBUG.TKEEP")) -> (s? t:f=w272:u8)
        n151 = Select(t=poc.ip.debug.states."Write.Data", s=w271, f=poc.ip.debug.states."Wait") -> (s? t:f=w282:T13)
      }
      frame "Write.Data" {
        # "arr"
        # "tkeep"
        # "tdata"
        # "state"
        # "tlast"
        # "tvalid"
        # "index"
        # "Write Packet Data"
        n152 = case shown="True" w286 {
          tunnel: w294 -> [w297 w303]
          tunnel: [w295 w312] -> w293
          tunnel: [TRUE w301] -> w291
          tunnel: [w297 w304] -> w290
          tunnel: [w299 w306] -> w289
          tunnel: [poc.ip.debug.states."Write.Data" w311] -> w288
          tunnel: w287 -> [w296 w307]
          tunnel: w285 -> [w299 _]
          tunnel: [w296 w307] -> w284
          tunnel: w283 -> [w295 _]
          frame False {
            # "index"
            # "arr"
            # "TDATA"
          }
          frame True {
            # "arr[3]"
            n153 = Index Array(array=w307, index=w303) -> (element=w312:u64)
            n154 = Increment(x=w303) -> (x+1=w304:u8)
            n155 = Equal?(x=u8 4, y=w303) -> (x = y?=w302:bool)
            n156 = Select(t=poc.ip.debug.states."Wait", s=w302, f=poc.ip.debug.states."Write.Data") -> (s? t:f=w311:T13)
            n157 = Not(x=w302) -> (.not. x?=w301:bool)
            n158 = Equal?(x=u8 3, y=w303) -> (x = y?=w306:bool)
          }
        }
      }
    }
    "MDEBUG.TDATA" <- w149
    "MDEBUG.TKEEP" <- w168
    "MDEBUG.TVALID" <- w167
    "MDEBUG.TLAST" <- w150
    n159 = xnode "Reset Register"("Register In"=w159) -> ("Data"=w158:u64)  [unwired: 1 out]
    n160 = Bundle By Name(cluster=w160, "state"=w188, "ob.cmd"=w185, "index"=w186, "TLAST"=w145, "TDATA"=w144) -> (w187:T17)
    n161 = Bundle By Name(cluster=w147, "state"=w138, "arr"=w136, "index"=w134, "TLAST"=w139, "TDATA"=w137) -> (w146:T18)
    n162 = Bundle By Name(cluster=w154, "state"=w153, "arr"=w152, "index"=w151, "TLAST"=w150, "TDATA"=w149) -> (w148:T18)
    n163 = Select(t=w154, s=w161, f=w148) -> (s? t:f=w166:T18)
    n164 = feedback-in #11(w166) -> ()
    n165 = Select(t=w160, s=w161, f=w187) -> (s? t:f=w184:T17)
    n166 = feedback-in #9(w184) -> ()
    n167 = Select(t=w147, s=w161, f=w146) -> (s? t:f=w190:T18)
    n168 = feedback-in #10(w190) -> ()
    n169 = disable-structure shown="FPGA_EMULATION==TRUE" {
      disable-tunnel: w140 -> [w440 _]
      disable-tunnel: w137 -> [w439 _]
      frame condition #0 (active) {
        w441 = cluster{"state":T14, "packet":u64[], "i":u16} {"state"=enum."Wait", "packet"=[0, 0, 0, 0], "i"=0}  # state
        # "TVALID"
        # "TDATA"
        # "For Testing"
        n170 = Bundle By Name(cluster=w441, "state"=poc.ip.axi.write.states."Wait" ("Enum")) -> (w445:cluster{"state":T14, "packet":u64[], "i":u16})
        n171 = feedback #12(w445) -> (w446:cluster{"state":T14, "packet":u64[], "i":u16})
        n172 = Unbundle By Name(w446) -> ("packet"=w451:u64[], "state"=w442:T14, "i"=w450:u16)
        n173 = case shown="\"Collect\"" w442 {
          tunnel: [FALSE w467] -> w443
          tunnel: [w453 w466] -> w448
          tunnel: w440 -> [w455 w463]
          tunnel: w439 -> [w458 w473]
          tunnel: [u16 1 ("i") w462] -> w449
          tunnel: [w457 w471] -> w452
          tunnel: w450 -> [_ w464]
          tunnel: w451 -> [_ w472]
          frame "Wait", Default {
            n174 = Replace Array Subset(array=u64[] [0, 0, 0, 0] ("packet"), new element=w458) -> (w457:u64[])  [unwired: 1 in]
            n175 = Select(t=poc.ip.axi.write.states."Collect" ("state"), s=w455, f=poc.ip.axi.write.states."Wait" ("state")) -> (s? t:f=w453:T14)
          }
          frame "Collect" {
            n176 = Replace Array Subset(array=w472, new element=w473, index=w464) -> (w471:u64[])
            n177 = Increment(x=w464) -> (x+1=w465:u16)
            n178 = Select(t=w465, s=w463, f=w464) -> (s? t:f=w462:u16)
            n179 = Equal?(x=u16 4, y=w462) -> (x = y?=w467:bool)
            n180 = Select(t=poc.ip.axi.write.states."Wait" ("Enum"), s=w467, f=poc.ip.axi.write.states."Collect" ("Enum")) -> (s? t:f=w466:T14)
          }
        }
        n181 = Bundle By Name(cluster=w446, "state"=w448, "packet"=w452, "i"=w449) -> (w447:cluster{"state":T14, "packet":u64[], "i":u16})
        n182 = feedback-in #12(w447) -> ()
        n183 = xnode "FIFO Write Using Handshaking"("Element"=w452, "Input Valid"=w443) -> ()  [unwired: 1 in, 2 out]
      }
      frame condition #1 {
      }
    }
    n184 = disable-structure shown="FPGA_EMULATION==TRUE" {
      disable-tunnel: w178 -> [w314 _]
      disable-tunnel: w144 -> [w313 _]
      frame condition #0 (active) {
        w315 = cluster{"state":T14, "packet":u64[], "i":u16} {"state"=enum."Wait", "packet"=[0, 0, 0, 0, 0, 0, 0, 0, 0, 0, 0, 0, 0, 0, 0, 0], "i"=0}  # state
        # "TVALID"
        # "TDATA"
        # "For Testing"
        n185 = Bundle By Name(cluster=w315, "state"=poc.ip.axi.write.states."Wait" ("Enum")) -> (w319:cluster{"state":T14, "packet":u64[], "i":u16})
        n186 = feedback #13(w319) -> (w320:cluster{"state":T14, "packet":u64[], "i":u16})
        n187 = Unbundle By Name(w320) -> ("packet"=w325:u64[], "state"=w316:T14, "i"=w324:u16)
        n188 = case shown="\"Wait\", Default" w316 {
          tunnel: [FALSE w341] -> w317
          tunnel: [w327 w340] -> w322
          tunnel: w314 -> [w329 w337]
          tunnel: w313 -> [w332 w347]
          tunnel: [u16 1 ("i") w336] -> w323
          tunnel: [w331 w345] -> w326
          tunnel: w324 -> [_ w338]
          tunnel: w325 -> [_ w346]
          frame "Wait", Default {
            n189 = Replace Array Subset(array=u64[] [0, 0, 0, 0, 0, 0, 0, 0, 0, 0, 0, 0, 0, 0, 0, 0] ("packet"), new element=w332) -> (w331:u64[])  [unwired: 1 in]
            n190 = Select(t=poc.ip.axi.write.states."Collect" ("state"), s=w329, f=poc.ip.axi.write.states."Wait" ("state")) -> (s? t:f=w327:T14)
          }
          frame "Collect" {
            n191 = Replace Array Subset(array=w346, new element=w347, index=w338) -> (w345:u64[])
            n192 = Increment(x=w338) -> (x+1=w339:u16)
            n193 = Select(t=w339, s=w337, f=w338) -> (s? t:f=w336:u16)
            n194 = Equal?(x=u16 16, y=w336) -> (x = y?=w341:bool)
            n195 = Select(t=poc.ip.axi.write.states."Wait" ("Enum"), s=w341, f=poc.ip.axi.write.states."Collect" ("Enum")) -> (s? t:f=w340:T14)
          }
        }
        n196 = Bundle By Name(cluster=w320, "state"=w322, "packet"=w326, "i"=w323) -> (w321:cluster{"state":T14, "packet":u64[], "i":u16})
        n197 = feedback-in #13(w321) -> ()
        n198 = xnode "FIFO Write Using Handshaking"("Element"=w326, "Input Valid"=w317) -> ()  [unwired: 1 in, 2 out]
      }
      frame condition #1 {
      }
    }
    n199 = disable-structure shown="FPGA_EMULATION==TRUE" {
      disable-tunnel: w167 -> [w236 _]
      disable-tunnel: w149 -> [w235 _]
      frame condition #0 (active) {
        w237 = cluster{"state":T14, "packet":u64[], "i":u16} {"state"=enum."Wait", "packet"=[0, 0, 0, 0], "i"=0}  # state
        # "TVALID"
        # "TDATA"
        # "For Testing"
        n200 = Bundle By Name(cluster=w237, "state"=poc.ip.axi.write.states."Wait" ("Enum")) -> (w241:cluster{"state":T14, "packet":u64[], "i":u16})
        n201 = feedback #14(w241) -> (w242:cluster{"state":T14, "packet":u64[], "i":u16})
        n202 = Unbundle By Name(w242) -> ("packet"=w247:u64[], "state"=w238:T14, "i"=w246:u16)
        n203 = case shown="\"Collect\"" w238 {
          tunnel: [FALSE w263] -> w239
          tunnel: [w249 w262] -> w244
          tunnel: w236 -> [w251 w259]
          tunnel: w235 -> [w254 w269]
          tunnel: [u16 1 ("i") w258] -> w245
          tunnel: [w253 w267] -> w248
          tunnel: w246 -> [_ w260]
          tunnel: w247 -> [_ w268]
          frame "Wait", Default {
            n204 = Replace Array Subset(array=u64[] [0, 0, 0, 0] ("packet"), new element=w254) -> (w253:u64[])  [unwired: 1 in]
            n205 = Select(t=poc.ip.axi.write.states."Collect" ("state"), s=w251, f=poc.ip.axi.write.states."Wait" ("state")) -> (s? t:f=w249:T14)
          }
          frame "Collect" {
            n206 = Replace Array Subset(array=w268, new element=w269, index=w260) -> (w267:u64[])
            n207 = Increment(x=w260) -> (x+1=w261:u16)
            n208 = Select(t=w261, s=w259, f=w260) -> (s? t:f=w258:u16)
            n209 = Equal?(x=u16 4, y=w258) -> (x = y?=w263:bool)
            n210 = Select(t=poc.ip.axi.write.states."Wait" ("Enum"), s=w263, f=poc.ip.axi.write.states."Collect" ("Enum")) -> (s? t:f=w262:T14)
          }
        }
        n211 = Bundle By Name(cluster=w242, "state"=w244, "packet"=w248, "i"=w245) -> (w243:cluster{"state":T14, "packet":u64[], "i":u16})
        n212 = feedback-in #14(w243) -> ()
        n213 = xnode "FIFO Write Using Handshaking"("Element"=w248, "Input Valid"=w239) -> ()  [unwired: 1 in, 2 out]
      }
      frame condition #1 {
      }
    }
    n214 = xnode "FIFO Read Using Handshaking"("Ready for Output"=TRUE, "FIFO In"=w174) -> ("Element"=w171:T21, "Output Valid"=w172:bool)  [unwired: 1 out]
    n215 = Select(t=w171, s=w172, f=w169) -> (s? t:f=w170:T6)
    n216 = call "bats.parser.vi"("time"=w158, "data.stream"=w170, "reset"=w161) -> ()  [unwired: 8 in, 1 out]
  }
  n217 = node-c288(w8) -> ()
  n218 = node-c288(w5) -> ()
